vi "Write FPGA_Ctl.vi"(8 "error in (no error)":errorcluster, 10 "FPGA_Ctl":cluster{"Mod":T1, "Span":sgl, "f0":sgl} {"f0" format="%#.3g"}, 11 "PAS Cell in":refnum<class "PAS Cell.lvclass">) -> (0 "error out":errorcluster, 3 "PAS Cell out":refnum<class "PAS Cell.lvclass">)   [LabVIEW 2015, in "PAS Cell.lvclass"]
uses:
  PAS Cell.lvclass
  Main/Controls/Laser Modulation.ctl
  PAS Cell.lvclass/PAS Cell.ctl
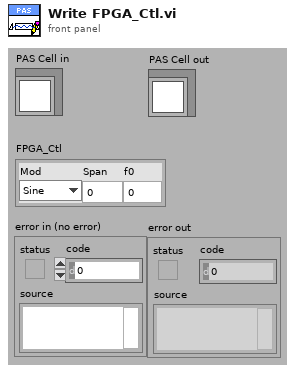
[diagram p1: front panel]
types:
  T1 = typedef "Laser Modulation.ctl" = enum8{"Sine", "Square"}
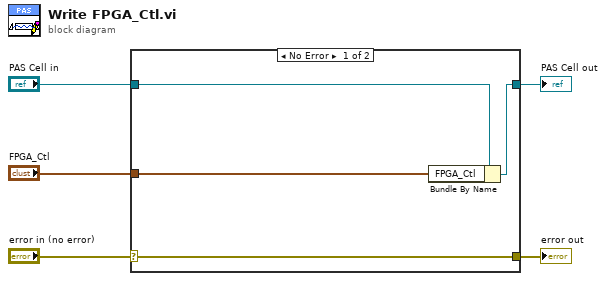
[diagram p0: block diagram]
diagram:
  n1 = case shown="No Error" "error in (no error)" {
    selector: "error in (no error)" -> [w9 w10]
    tunnel: [w9 w10] -> w4
    tunnel: [w7 w11] -> w2
    tunnel: "PAS Cell in" -> [w8 w11]
    tunnel: "FPGA_Ctl" -> [w6 _]
    frame No Error {
      n2 = Bundle By Name(cluster=w8, "FPGA_Ctl"=w6) -> (w7:refnum<class "PAS Cell.lvclass">)
    }
    frame Error {
    }
  }
  "error out" <- w4
  "PAS Cell out" <- w2
